vi "Delete Many Attributes.vi"(7 "Unique ID":string, 8 "error in (no error)":errorcluster, 9 "Types":variant[](array[variant]), 10 "Attribute Names":string[](array[string]), 11 "Linked List in":refnum<class "Linked List.lvclass">) -> (0 "error out":errorcluster, 1 "Found?":bool, 3 "Linked List out":refnum<class "Linked List.lvclass">)   [LabVIEW 2020, in "Linked Lists.lvlib" / "Linked List.lvclass"]
uses:
  <vilib>/gpm_packages/@cs/linked-list/Source/Linked List/Linked List/Linked List.lvclass
  <vilib>/gpm_packages/@cs/linked-list/Source/Linked List/Linked List Definition/Linked List Definition.lvclass
  <vilib>/gpm_packages/@cs/linked-list/Source/Linked List/Linked List/Linked List.lvclass/Linked List.ctl
  <vilib>/gpm_packages/@cs/lookup-table/Source/LookupTable/LookupTable.lvclass/LookupTable.ctl
  beab1386-fb03-4602-991d-c6dd99164584.vi
  fefba692-d654-4111-87d6-35e0be03b322.vi
  c3a41b57-1de6-40c5-b62f-7afd20616e25.vi
  28e376cc-0c53-4ad0-9646-dabd36273828.vi
  <vilib>/gpm_packages/@cs/lookup-table/Source/LookupTable/Read Table Reference.vi
  beab1386-fb03-4602-991d-c6dd99164584.vi/7de3be9f-c4e8-4fe0-b5c9-025b0e8f7ec2.vi
  28e376cc-0c53-4ad0-9646-dabd36273828.vi/3ea1e12b-1e2c-4722-8490-afdc728592de.vi
  <vilib>/gpm_packages/@cs/lookup-table/Source/LookupTable/LookupTable.lvclass
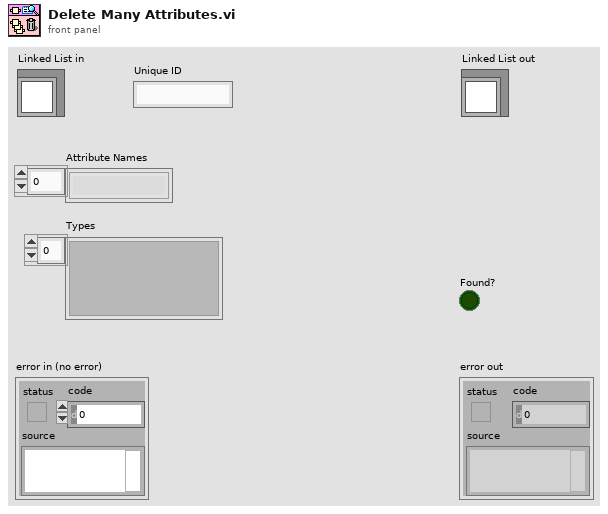
[diagram p1: front panel]
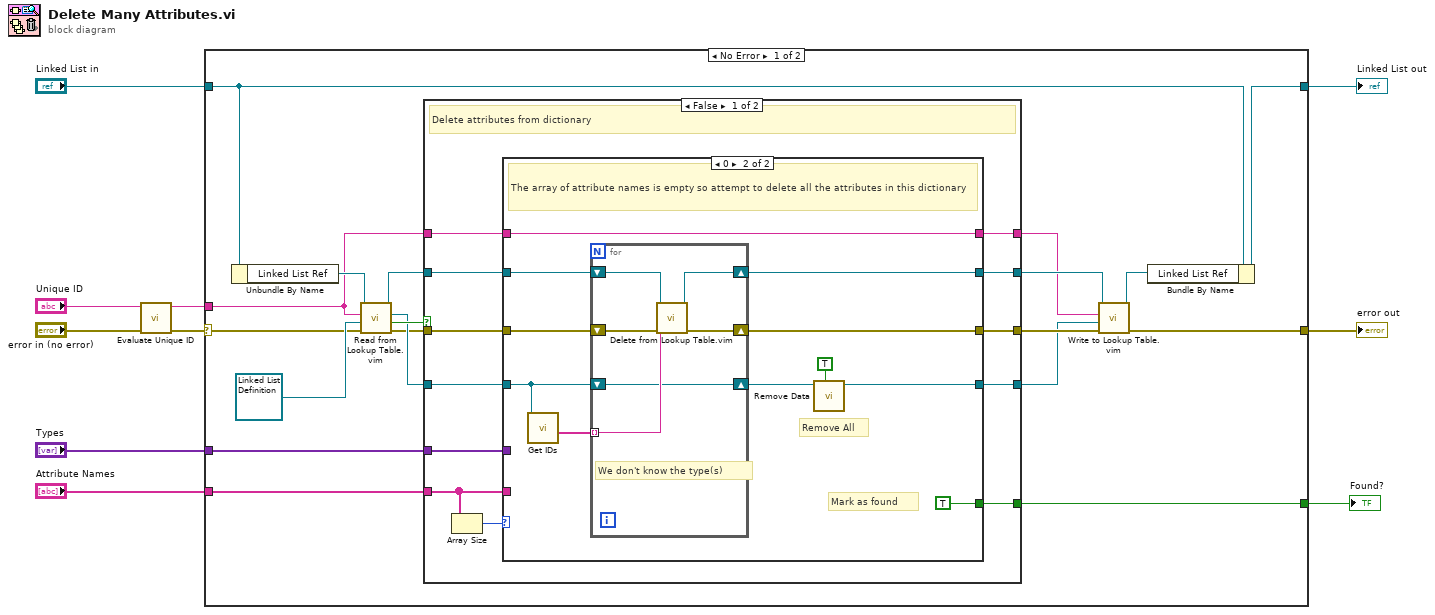
[diagram p0: block diagram]
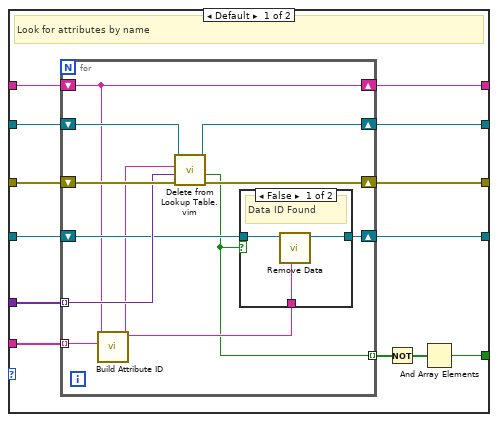
[diagram p2: hidden frame]
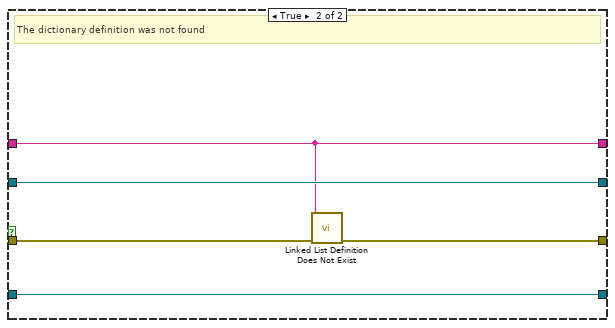
[diagram p4: hidden frame]
diagram:
  n1 = call <vilib>:"Evaluate Unique ID.vi"("error in (no error)"="error in (no error)", "Unique ID"="Unique ID") -> ("error out"=w7:errorcluster, "Unique ID Out"=w5:string)  [unwired: 8 in]
  n2 = case shown="No Error" w7 {
    selector: w7 -> [w21 w92]
    tunnel: [w22 w93] -> w8
    tunnel: "Linked List in" -> [w23 w93]
    tunnel: w5 -> [w20 _]
    tunnel: [w15 w92] -> w4
    tunnel: "Attribute Names" -> [w19 _]
    tunnel: "Types" -> [w18 _]
    tunnel: [w11 _] -> w1
    frame No Error {
      n3 = Unbundle By Name(w23) -> ("Linked List Ref"=w29:refnum<data-value>)
      n4 = call "Read from Lookup Table.vim"("error in (no error)"=w21, "Type"=refnum<class "Linked List Definition.lvclass"> refnum ("Linked List.lvlib:Linked List Definition.lvclass"), "Item Name"=w20, "LookupTable Reference"=w29) -> ("error out"=w24:errorcluster, "Not Found?"=w27:bool, "Value"=w25:refnum<class "Linked List Definition.lvclass">, "LookupTable Reference Out"=w26:refnum<data-value>)  [unwired: 4 in]
      n5 = case shown="False" w27 {
        tunnel: w26 -> [w40 w89]
        tunnel: w25 -> [w38 w87]
        tunnel: [w37 w90] -> w14
        tunnel: w24 -> [w41 w91]
        tunnel: w20 -> [w39 w88]
        tunnel: [w36 w89] -> w16
        tunnel: w19 -> [w35 _]
        tunnel: w18 -> [w33 _]
        tunnel: [w32 w87] -> w12
        tunnel: [w31 w88] -> w13
        tunnel: [w30 _] -> w11
        frame False {
          # "Delete attributes from dictionary"
          n6 = Array Size(array=w35) -> (size(s)=w34:i32)
          n7 = case shown="0" w34 {
            tunnel: w41 -> [w52 w80]
            tunnel: w40 -> [w54 w79]
            tunnel: w39 -> [w49 w71]
            tunnel: w38 -> [w47 w75]
            tunnel: [w51 w78] -> w37
            tunnel: [w53 w77] -> w36
            tunnel: w35 -> [w50 _]
            tunnel: w33 -> [w48 _]
            tunnel: [w46 w73] -> w32
            tunnel: [w45 w71] -> w31
            tunnel: [w43 TRUE] -> w30
            frame Default {
              # "Look for attributes by name"
              n8 = for {
                shift-right: [w61] -> w53
                shift-left: w54 -> [w62]
                shift-right: [w63] -> w51
                shift-left: w52 -> [w64]
                tunnel: w50 -> [w65] mode=indexing
                tunnel: w48 -> [w60] mode=indexing
                shift-right: [w58] -> w46
                shift-left: w47 -> [w59]
                shift-right: [w56] -> w45
                shift-left: w49 -> [w56]
                tunnel: [w55] -> w44 mode=indexing
                n9 = call <vilib>:"Build Attribute ID.vi"("Attr Name"=w65, "Unique ID"=w56) -> ("Attr ID Out"=w57:string)  [unwired: 9 in]
                n10 = call "Delete from Lookup Table.vim"("error in (no error)"=w64, "Confirm Type"=w60, "Item Name"=w57, "LookupTable Reference"=w62) -> ("error out"=w63:errorcluster, "Not Found?"=w55:bool, "LookupTable Reference Out"=w61:refnum<data-value>)  [unwired: 5 in]
                n11 = case shown="False" w55 {
                  tunnel: w59 -> [w68 w69]
                  tunnel: [w67 w69] -> w58
                  tunnel: w57 -> [w66 _]
                  frame False {
                    # "Data ID Found"
                    n12 = call <vilib>:"Remove Data.vi"("Unique ID"=w66, "Linked List Definition in"=w68) -> ("Linked List Definition out"=w67:refnum<class "Linked List Definition.lvclass">)  [unwired: 9 in]
                  }
                  frame True {
                    # "Data ID not found"
                  }
                }
              }
              n13 = Not(x=w44) -> (.not. x?=w42:bool[])
              n14 = And Array Elements(Boolean array=w42) -> (logical AND=w43:bool)
            }
            frame 0 {
              # "Mark as found"
              # "Remove All"
              # "The array of attribute names is empty so attempt to delete all the attributes in this dictionary"
              n15 = call <vilib>:"Get IDs.vi"("Linked List Definition in"=w75) -> ("Data IDs"=w76:string[])  [unwired: 8 in, 2 out]
              n16 = for {
                shift-right: [w83] -> w78
                shift-left: w80 -> [w84]
                shift-right: [w85] -> w77
                shift-left: w79 -> [w86]
                tunnel: w76 -> [w82] mode=indexing
                shift-right: [w81] -> w74
                shift-left: w75 -> [w81]
                # "We don't know the type(s)"
                n17 = call "Delete from Lookup Table.vim"("error in (no error)"=w84, "Item Name"=w82, "LookupTable Reference"=w86) -> ("error out"=w83:errorcluster, "LookupTable Reference Out"=w85:refnum<data-value>)  [unwired: 6 in, 1 out]
              }
              n18 = call <vilib>:"Remove Data.vi"("Remove All?"=TRUE, "Linked List Definition in"=w74) -> ("Linked List Definition out"=w73:refnum<class "Linked List Definition.lvclass">)  [unwired: 9 in]
            }
          }
        }
        frame True {
          # "The dictionary definition was not found"
          n19 = call <vilib>:"Linked List Definition Does Not Exist.vi"("Error In"=w91, "Unique ID"=w88) -> ("Error Out"=w90:errorcluster)  [unwired: 9 in]
        }
      }
      n20 = call "Write to Lookup Table.vim"("error in (no error)"=w14, "Item"=w12, "Item Name"=w13, "LookupTable Reference"=w16) -> ("error out"=w15:errorcluster, "LookupTable Reference Out"=w17:refnum<data-value>)  [unwired: 5 in, 1 out]
      n21 = Bundle By Name(cluster=w23, "Linked List Ref"=w17) -> (w22:refnum<class "Linked List.lvclass">)
    }
    frame Error {
    }
  }
  "error out" <- w4
  "Linked List out" <- w8
  "Found?" <- w1
